vi "Initialize From Config.vi"(8 "error in":errorcluster, 9 "Module Configurations":refnum<class "TBM module configuration.lvclass">[](array[class]), 10 "Modules":refnum<class "TBM module execution interface.lvclass">[](array[class]), 11 "Engine Configuration":refnum<class "synchronous engine configuration.lvclass">) -> (0 "error out":errorcluster, 3 "Engine Data Out":T1={"Main Tag Data"={"Double"=[], "Single"=[], "I64"=[], "I32"=[], "I16"=[], "I8"=[], "U64"=[], "U32"=[], "U16"=[], "U8"=[], "Boolean"=[], "String"=[], "Array of Double"=[], "Array of Single"=[], "Array of I64"=[], "Array of I32"=[], "Array of I16"=[], "Array of I8"=[], "Array of U64"=[], "Array of U32"=[], "Array of U16"=[], "Array of U8"=[], "Array of Boolean"=[], "Array of String"=[]}, "Module Info"={"Tag Bus Modules"=[], "Input Method Indices"=[], "Process Method Indices"=[], "Output Method Indices"=[], "Input Transfer Specifications"=[], "Parameter Transfer Specifications"=[], "Result Transfer Specifications"=[], "Output Transfer Specifications"=[], "Module Errors"=[], "UID"=""}, "Safe State?"=FALSE, "engine timing source"=refnum, "Processor"=5000, "Priority"=-2})   [LabVIEW 2013, in "synchronous engine runtime.lvclass"]
uses:
  synchronous engine runtime.lvclass
  Engine Data.ctl
  <vilib>/NI/Module Timing Source/timing source/TBM timing source.lvclass
  <vilib>/NI/Tag Bus/table/data table.ctl
  Module Execution Info.ctl
  <vilib>/NI/Tag Bus Module Framework/runtime/TBM module execution interface.lvclass
  Data Table with Transfer Spec.ctl
  <vilib>/NI/Tag Bus/table/transfer specification.ctl
  <vilib>/NI/Tag Bus/tag/Data Type.ctl
  Configuration/synchronous engine configuration.lvclass
  <vilib>/NI/Tag Bus Module Framework/module configuration/TBM module configuration.lvclass
  <vilib>/NI/Module Timing Source/usec timing source/usec timing source.lvclass
  Configuration/synchronous engine configuration.lvclass/synchronous engine configuration.ctl
  Engine Configuration/engine configuration.lvclass/engine configuration.ctl
  <vilib>/NI/Module Timing Source/timing source/TBM timing source.lvclass/TBM timing source.ctl
  <vilib>/NI/Tag Bus/dictionary/data dictionary.lvclass/data dictionary.ctl
  <vilib>/NI/CEF/CEF_TreeControl/serializable configuration/NISE_CEF_serializable configuration.lvclass/NISE_CEF_serializable configuration.ctl
  <vilib>/NI/CEF/CEF_TreeControl/serializable configuration/NISE_CEF_serializable configuration.lvclass
  <vilib>/NI/CEF/CEF_TreeControl/serializable configuration/Read UID.vi
  Configuration/Read Processor.vi
  Configuration/Read Priority.vi
  Configuration/Read Timing Source dt.vi
  <vilib>/NI/Tag Bus/dictionary/data dictionary.lvclass
  Engine Configuration/engine configuration.lvclass
  <vilib>/NI/Tag Bus/table/data table.lvlib
  <vilib>/NI/Tag Bus/tag/tag descriptor.lvclass
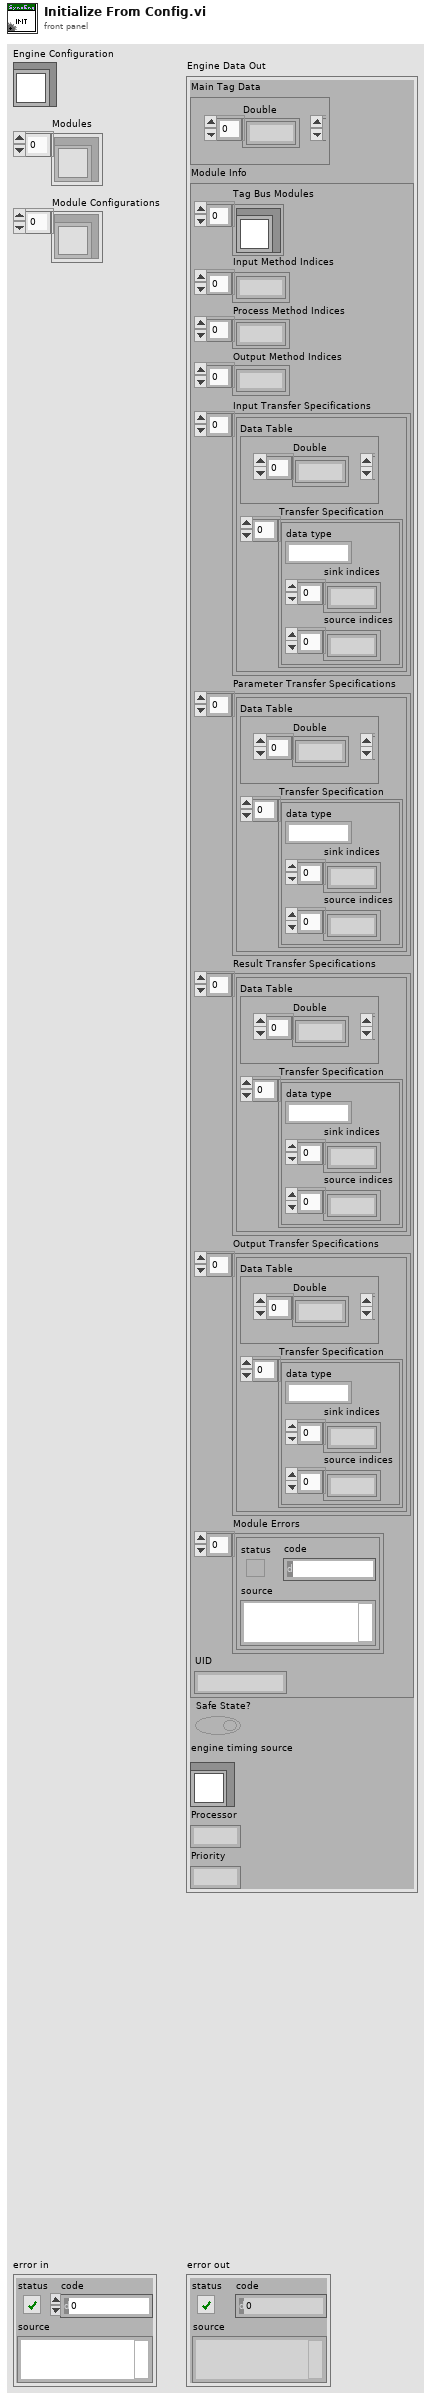
[diagram p1: front panel]
types:
  T1 = typedef "synchronous engine runtime.lvclass/Engine Data.ctl" = cluster{"Main Tag Data":T2, "Module Info":T3, "Safe State?":bool, "engine timing source":refnum<class "TBM timing source.lvclass">, "Processor":i32, "Priority":i32}
  T2 = typedef "tag bus.lvlib/data table.lvlib/data table.ctl" = cluster{"Double":dbl[], "Single":sgl[], "I64":i64[], "I32":i32[], "I16":i16[], "I8":i8[], "U64":u64[], "U32":u32[], "U16":u16[], "U8":u8[], "Boolean":bool[], "String":string[], "Array of Double":cluster{"DBL Array":dbl[]}[], "Array of Single":cluster{"SGL Array":sgl[]}[], "Array of I64":cluster{"I64 Array":i64[]}[], "Array of I32":cluster{"I32 Array":i32[]}[], "Array of I16":cluster{"I16 Array":i16[]}[], "Array of I8":cluster{"I8 Array":i8[]}[], "Array of U64":cluster{"U64 Array":u64[]}[], "Array of U32":cluster{"U32 Array":u32[]}[], "Array of U16":cluster{"U16 Array":u16[]}[], "Array of U8":cluster{"U8 Array":u8[]}[], "Array of Boolean":cluster{"Boolean Array":bool[]}[], "Array of String":cluster{"String Array":string[]}[]}
  T3 = typedef "synchronous engine runtime.lvclass/Module Execution Info.ctl" = cluster{"Tag Bus Modules":refnum<class "TBM module execution interface.lvclass">[], "Input Method Indices":i32[], "Process Method Indices":i32[], "Output Method Indices":i32[], "Input Transfer Specifications":T4[], "Parameter Transfer Specifications":T4[], "Result Transfer Specifications":T4[], "Output Transfer Specifications":T4[], "Module Errors":errorcluster[], "UID":string}
  T4 = typedef "synchronous engine runtime.lvclass/Data Table with Transfer Spec.ctl" = cluster{"Data Table":T2, "Transfer Specification":T5[]}
  T5 = typedef "tag bus.lvlib/data table.lvlib/transfer specification.ctl" = cluster{"data type":T6, "sink indices":i32[], "source indices":i32[]}
  T6 = typedef "tag bus.lvlib/tag descriptor.lvclass/Data Type.ctl" = enum16{"Double", "Single", "I64", "I32", "I16", "I8", "U64", "U32", "U16", "U8", "Boolean", "String", "Array of Double", "Array of Single", "Array of I64", "Array of I32", "Array of I16", "Array of I8", "Array of U64", "Array of U32", "Array of U16", "Array of U8", "Array of Boolean", "Array of String"}
  T7 = typedef "TBM channel.lvclass/data tables.ctl" = cluster{"input data":T8, "processing parameter":T8, "processing result":T8, "output data":T8}
  T8 = typedef "tag bus.lvlib/dictionary table pair.ctl" = cluster{"data dictionary":refnum<class "data dictionary.lvclass">, "data table":T2}
  T9 = typedef "TBM module execution interface.lvclass/execution settings.ctl" = cluster{"reads inputs":bool, "processes data":bool, "writes outputs":bool}
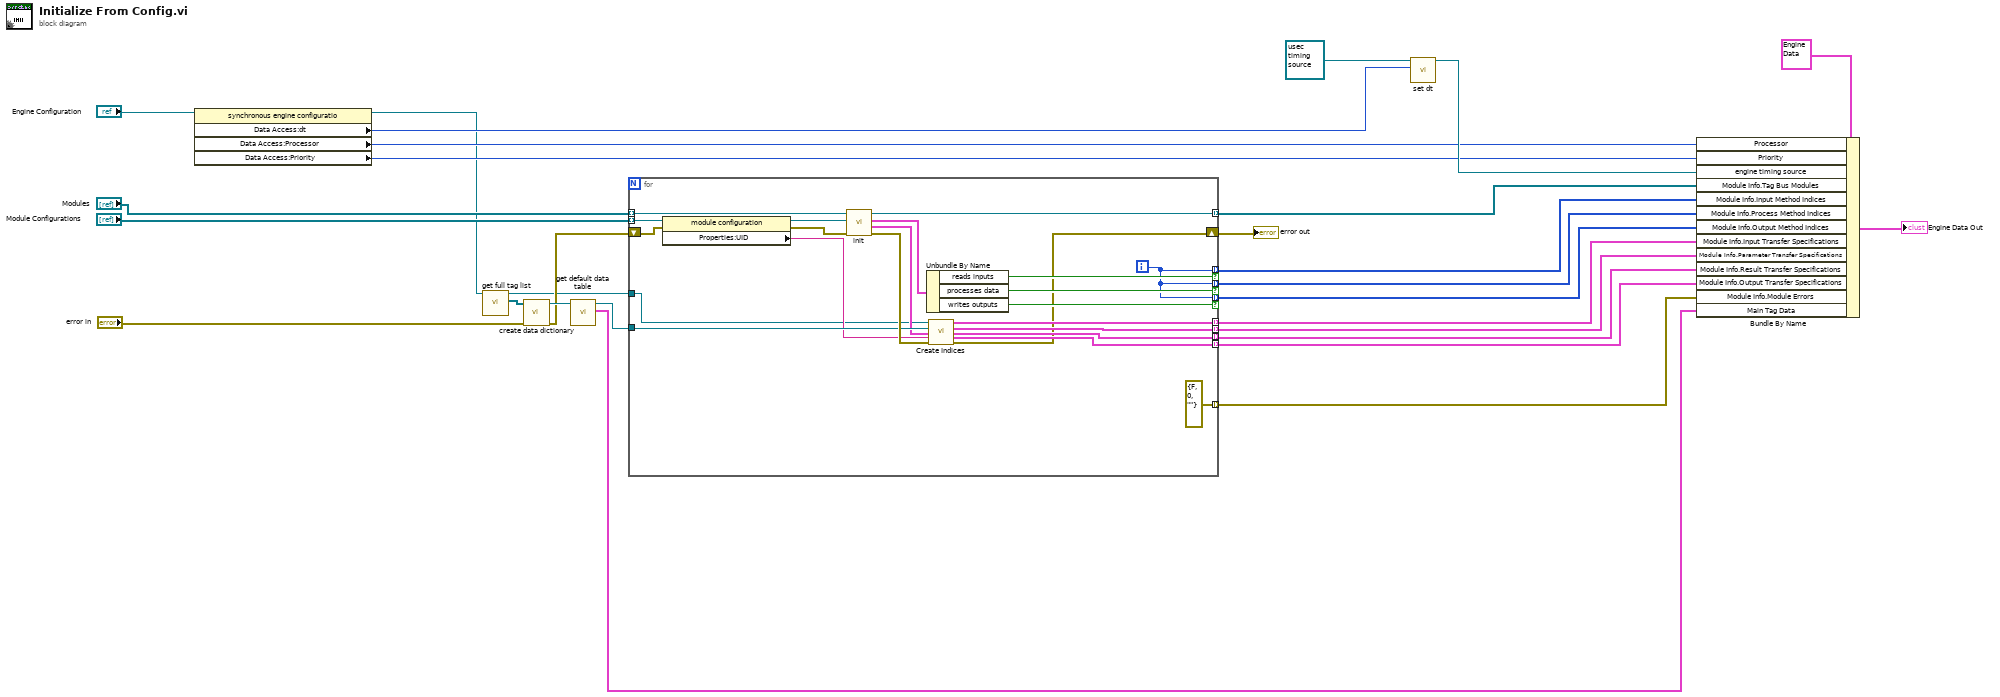
[diagram p0: block diagram]
diagram:
  n1 = property class="synchronous engine configuratio"(reference="Engine Configuration") -> (reference out=w1:refnum<class "synchronous engine configuration.lvclass">, "Data Access:dt"=w4:u32, "Data Access:Processor"=w3:i32, "Data Access:Priority"=w2:i32)  [unwired: 1 in, 1 out]
  n2 = call "get full tag list.vi"("engine configuration in"=w1) -> ("tag list"=w11:refnum<class "tag descriptor.lvclass">[], "engine configuration out"=w8:refnum<class "synchronous engine configuration.lvclass">)  [unwired: 9 in]
  n3 = call <vilib>:"create data dictionary.vi"("error in"="error in", "system tags"=w11) -> ("error out"=w9:errorcluster, "data dictionary"=w10:refnum<class "data dictionary.lvclass">)  [unwired: 8 in]
  n4 = call <vilib>:"get default data table.vi"("data dictionary in"=w10) -> ("default data table"=w17:T2, "data dictionary out"=w16:refnum<class "data dictionary.lvclass">)  [unwired: 9 in]
  n5 = for {
    tunnel: "Module Configurations" -> [w36] mode=indexing
    shift-right: [w31] -> w19
    shift-left: w9 -> [w33]
    tunnel: "Modules" -> [w50] mode=indexing
    tunnel: [w32] -> w28 mode=indexing
    tunnel: [w41] -> w26 mode=indexing if=w49
    tunnel: [w41] -> w25 mode=indexing if=w48
    tunnel: [w41] -> w24 mode=indexing if=w47
    tunnel: [w46] -> w23 mode=indexing
    tunnel: [w45] -> w22 mode=indexing
    tunnel: [w44] -> w21 mode=indexing
    tunnel: [w43] -> w20 mode=indexing
    tunnel: [errorcluster {"status"=FALSE, "code"=0, "source"=""} ("error constant")] -> w18 mode=indexing
    tunnel: w16 -> [w39]
    tunnel: w8 -> [w29]
    i -> [w41]
    n6 = property class="module configuration"(reference=w36, error in=w33) -> (reference out=w35:refnum<class "TBM module configuration.lvclass">, error out=w34:errorcluster, "Properties:UID"=w30:string)
    n7 = call-dynamic "init.vi"("error in"=w34, "module configuration"=w35, "module in"=w50) -> ("error out"=w42:errorcluster, "data allocations"=w37:T7, "execution settings"=w38:T9, "module out"=w32:refnum<class "TBM module execution interface.lvclass">)  [unwired: 5 in]
    n8 = Unbundle By Name(w38) -> ("reads inputs"=w49:bool, "processes data"=w48:bool, "writes outputs"=w47:bool)
    n9 = call "Create Indices.vi"("synchronous engine configuration"=w29, "main data dictionary"=w39, "data description"=w37, "Module ID"=w30, "error in"=w42) -> ("Input Transfer Specification"=w46:T4, "Parameter Transfer Specifcation"=w45:T4, "Result Transfer Specifcation"=w44:T4, "Output Transfer Specifcation"=w43:T4, "error out"=w31:errorcluster)  [unwired: 6 in]
  }
  "error out" <- w19
  n10 = call <vilib>:"set dt.vi"("dt"=w4, "timing source in"=refnum<class "usec timing source.lvclass"> refnum ("usec timing source.lvclass")) -> ("timing source out"=w5:refnum<class "usec timing source.lvclass">)  [unwired: 9 in]
  n11 = Bundle By Name(cluster=T1 {"Main Tag Data"={"Double"=[], "Single"=[], "I64"=[], "I32"=[], "I16"=[], "I8"=[], "U64"=[], "U32"=[], "U16"=[], "U8"=[], "Boolean"=[], "String"=[], "Array of Double"=[], "Array of Single"=[], "Array of I64"=[], "Array of I32"=[], "Array of I16"=[], "Array of I8"=[], "Array of U64"=[], "Array of U32"=[], "Array of U16"=[], "Array of U8"=[], "Array of Boolean"=[], "Array of String"=[]}, "Module Info"={"Tag Bus Modules"=[], "Input Method Indices"=[], "Process Method Indices"=[], "Output Method Indices"=[], "Input Transfer Specifications"=[], "Parameter Transfer Specifications"=[], "Result Transfer Specifications"=[], "Output Transfer Specifications"=[], "Module Errors"=[], "UID"=""}, "Safe State?"=FALSE, "engine timing source"=refnum, "Processor"=0, "Priority"=0} ("Engine Data"), "Processor"=w3, "Priority"=w2, "engine timing source"=w5, "Module Info.Tag Bus Modules"=w28, "Module Info.Input Method Indices"=w26, "Module Info.Process Method Indices"=w25, "Module Info.Output Method Indices"=w24, "Module Info.Input Transfer Specifications"=w23, "Module Info.Parameter Transfer Specifications"=w22, "Module Info.Result Transfer Specifications"=w21, "Module Info.Output Transfer Specifications"=w20, "Module Info.Module Errors"=w18, "Main Tag Data"=w17) -> (→"Engine Data Out":T1)
